vi "Temperature serial v6.vi"(0 "Command String":string, 5 "Time Out (S)":dbl, 7 "CALIB":dbl) -> (4 "T1":dbl, 6 "T2":dbl, 8 "T3":dbl, 10 "T4":dbl, 13 "error":bool, 14 "output cluster":cluster{dbl, dbl, dbl, dbl, i32, "error #":dbl}, 15 "Unit ID":dbl)   [LabVIEW 2013]
uses:
  program files/Global 1.vi
  <vilib>/Instr/_visa.llb/VISA Configure Serial Port (Instr).vi
panel:
  out "COM port":refnum<visa-resource-name>="COM6"
  out "error #":dbl
  out "End T":dbl
  out "Start T":dbl
  out "read time":dbl
  in  "Array - String":string[](array[string])
  out "end of data (#)":bool
  out "data bytes read":dbl
  out "data string":string
  out "read buffer":string
  out "error out":errorcluster
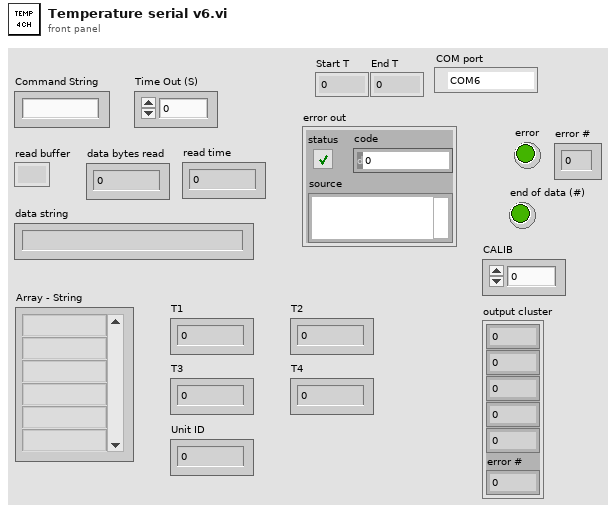
[diagram p1: front panel]
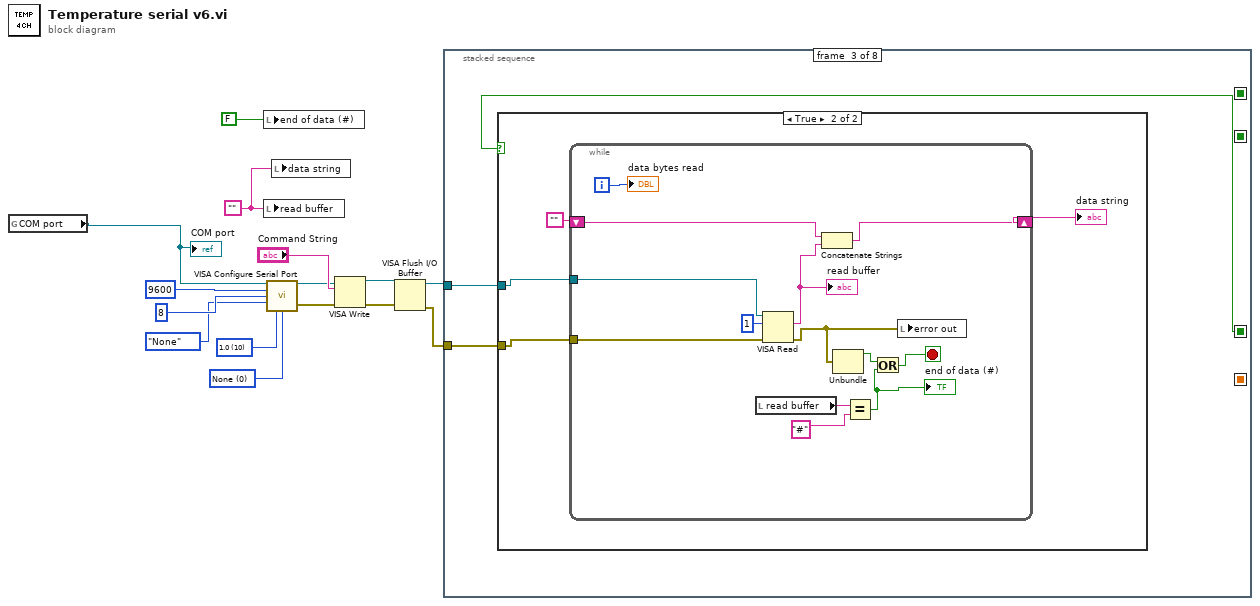
[diagram p0: block diagram]
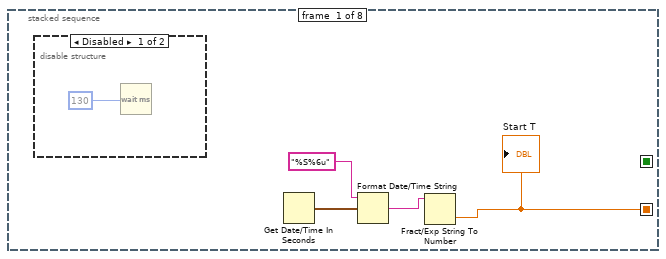
[diagram p2: hidden frame]
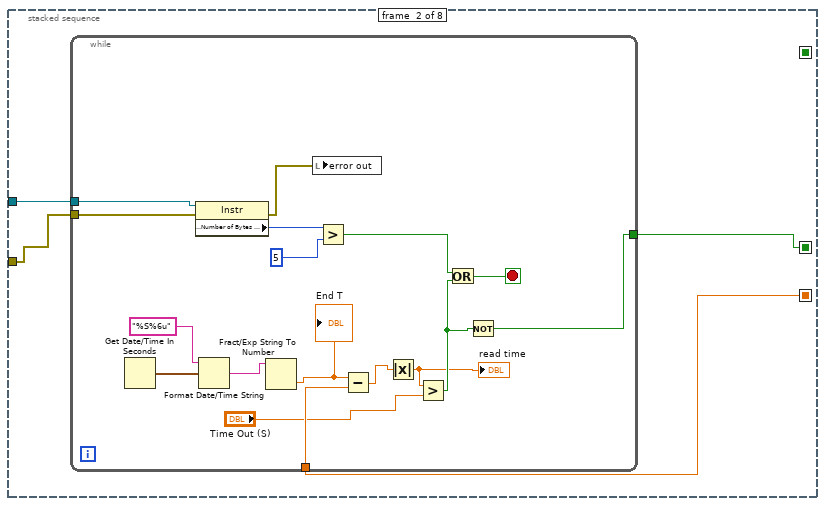
[diagram p4: hidden frame]
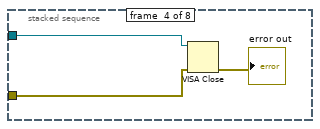
[diagram p6: hidden frame]
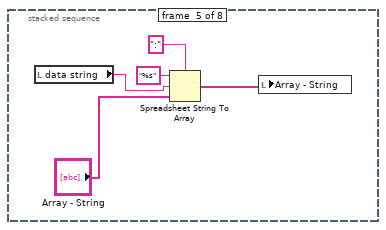
[diagram p7: hidden frame]
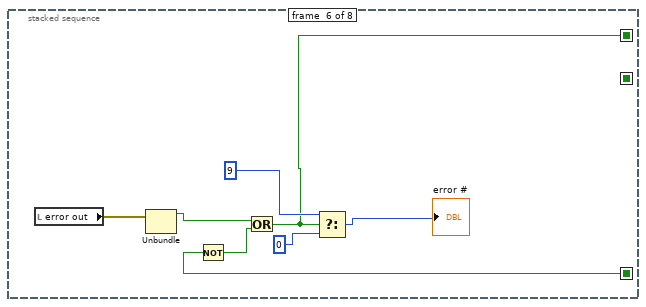
[diagram p8: hidden frame]
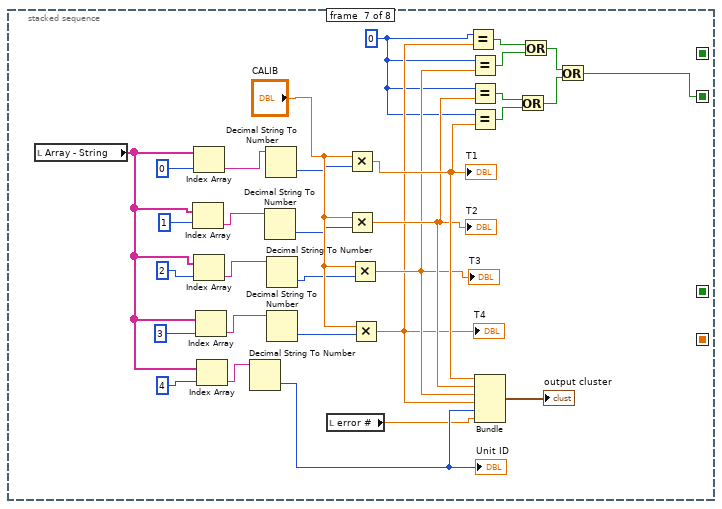
[diagram p9: hidden frame]
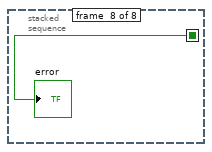
[diagram p10: hidden frame]
diagram:
  w2 = ""
  w11 = u16 0 items=["None", "XON/XOFF", "RTS/CTS", "XON/XOFF & RTS/CTS", "DTR/DSR", "XON/XOFF & DTR/DSR"] ("flow control (0:none)")
  w12 = u16 10 items=["1.0"=10, "1.5"=15, "2.0"=20] ("stop bits (10: 1 bit)")
  n1 = global read "Global 1.vi" "COM port"() -> (w1:refnum<visa-resource-name>)
  "COM port" <- w1
  n2 = local write "end of data (#)"(FALSE) -> ()
  n3 = local write "read buffer"(w2) -> ()
  n4 = call-poly "VISA Configure Serial Port"("VISA resource name"=w1, "baud rate (9600)"=u32 9600, "data bits (8)"=u16 8, "parity (0:none)"=enum16{"None", "Odd", "Even", "Mark", "Space"}."None", "stop bits (10: 1 bit)"=w12, "flow control (0:none)"=w11) -> ("VISA resource name out"=w4:refnum<visa-resource-name>, "error out"=w3:errorcluster)  [unwired: 8 in]
  n5 = local write "data string"(w2) -> ()
  n6 = VISA Write(VISA resource name=w4, write buffer="Command String", error in (no error)=w3) -> (VISA resource name out=w9:refnum<visa-resource-name>, error out=w8:errorcluster)  [unwired: 1 out]
  n7 = VISA Flush I/O Buffer(VISA resource name=w9, error in (no error)=w8) -> (VISA resource name out=w7:refnum<visa-resource-name>, error out=w6:errorcluster)  [unwired: 1 in]
  n8 = stacked-sequence {
    seq-local: [_ w22 _ _ _ _ _ _] -> [_ _ w42 _ _ w75 _ _]
    seq-local: [w16 _ _ _ _ _ _ _] -> [_ w21 _ _ _ _ _ _]
    seq-local: [_ _ _ _ _ w70 _ _] -> [_ _ _ _ _ _ _ _]
    seq-local: [_ _ _ _ _ _ w78 _] -> [_ _ _ _ _ _ _ w109]
    tunnel: w7 -> [_ w24 w44 w64 _ _ _ _]
    tunnel: w6 -> [_ w23 w43 w63 _ _ _ _]
    frame #0 {
      n9 = disable-structure shown="Disabled" {
        frame Disabled {
          n10 = Wait (ms)(milliseconds to wait=130) -> ()  [unwired: 1 out]
        }
        frame Enabled {
        }
      }
      n11 = Get Date/Time In Seconds() -> (seconds since 1Jan1904=w19:timestamp)
      n12 = Format Date/Time String(time format string (%c)="%S%6u", seconds (now)=w19) -> (date/time string=w17:string)  [unwired: 1 in]
      n13 = Fract/Exp String To Number(string=w17) -> (number=w16:dbl)  [unwired: 3 in, 1 out]
      "Start T" <- w16
    }
    frame #1 {
      n14 = while {
        tunnel: w24 -> [w41]
        tunnel: w23 -> [w40]
        tunnel: [w28] -> w22
        tunnel: w21 -> [w32]
        stop <- w30 stop-if-true
        n15 = Get Date/Time In Seconds() -> (seconds since 1Jan1904=w36:timestamp)
        n16 = property class="Instr"(reference=w41, error in=w40) -> (error out=w37:errorcluster, "Serial Settings:Number of Bytes at Serial Port"=w39:u32)  [unwired: 1 out]
        n17 = Format Date/Time String(time format string (%c)="%S%6u", seconds (now)=w36) -> (date/time string=w34:string)  [unwired: 1 in]
        n18 = Fract/Exp String To Number(string=w34) -> (number=w33:dbl)  [unwired: 3 in, 1 out]
        "End T" <- w33
        n19 = local write "error out"(w37) -> ()
        n20 = Greater?(x=w39, y=5) -> (0:w31:bool)
        n21 = Subtract(x=w33, y=w32) -> (x-y=w26:dbl)
        n22 = Absolute Value(x=w26) -> (abs(x)=w25:dbl)
        "read time" <- w25
        n23 = Greater?(x=w25, y="Time Out (S)") -> (0:w29:bool)
        n24 = Or(x=w31, y=w29) -> (x .or. y?=w30:bool)
        n25 = Not(x=w29) -> (.not. x?=w28:bool)
      }
    }
    frame #2 {
      n26 = case shown="True" w42 {
        tunnel: w44 -> [_ w48]
        tunnel: w43 -> [_ w47]
        frame False {
        }
        frame True {
          n27 = while {
            tunnel: w48 -> [w56]
            tunnel: w47 -> [w55]
            shift-right: [w54] -> w46
            shift-left: "" -> [w53]
            i -> [w57]
            stop <- w49 stop-if-true
            n28 = local read "read buffer"() -> (w60:string)
            n29 = VISA Read(VISA resource name=w56, byte count=u32 1, error in (no error)=w55) -> (read buffer=w58:string, error out=w52:errorcluster)  [unwired: 2 out]
            "read buffer" <- w58
            n30 = Concatenate Strings(w53, w58) -> (w54:string)
            n31 = Unbundle(w52) -> ("status"=w51:bool)  [unwired: 2 out]
            n32 = Equal?(x=w60, y="#") -> (x = y?=w50:bool)
            "end of data (#)" <- w50
            n33 = Or(x=w51, y=w50) -> (x .or. y?=w49:bool)
            n34 = local write "error out"(w52) -> ()
            "data bytes read" <- w57
          }
          "data string" <- w46
        }
      }
    }
    frame #3 {
      n35 = VISA Close(VISA resource name=w64, error in (no error)=w63) -> (error out=→"error out":errorcluster)
    }
    frame #4 {
      n36 = local read "data string"() -> (w67:string)
      n37 = Spreadsheet String To Array(delimiter (Tab)=":", format string="%s", spreadsheet string=w67, array type (2D Dbl)="Array - String") -> (array=w65:string[])
      n38 = local write "Array - String"(w65) -> ()
    }
    frame #5 {
      n39 = local read "error out"() -> (w77:errorcluster)
      n40 = Unbundle(w77) -> ("status"=w76:bool)  [unwired: 2 out]
      n41 = Not(x=w75) -> (.not. x?=w74:bool)
      n42 = Or(x=w76, y=w74) -> (x .or. y?=w70:bool)
      n43 = Select(t=9, s=w70, f=0) -> (s? t:f=→"error #":i32)
    }
    frame #6 {
      w85 = 0
      n44 = local read "Array - String"() -> (w100:string[])
      n45 = Index Array(array=w100, index=1) -> (element=w103:string)
      n46 = Index Array(array=w100, index=0) -> (element=w107:string)
      n47 = Index Array(array=w100, index=2) -> (element=w102:string)
      n48 = Index Array(array=w100, index=3) -> (element=w101:string)
      n49 = Index Array(array=w100, index=4) -> (element=w98:string)
      n50 = Decimal String To Number(string=w98) -> (number=w92:i32)  [unwired: 2 in, 1 out]
      "Unit ID" <- w92
      n51 = Decimal String To Number(string=w103) -> (number=w95:i32)  [unwired: 2 in, 1 out]
      n52 = Decimal String To Number(string=w107) -> (number=w96:i32)  [unwired: 2 in, 1 out]
      n53 = Decimal String To Number(string=w102) -> (number=w94:i32)  [unwired: 2 in, 1 out]
      n54 = Decimal String To Number(string=w101) -> (number=w93:i32)  [unwired: 2 in, 1 out]
      n55 = local read "error #"() -> (w91:dbl)
      n56 = Multiply(x="CALIB", y=w96) -> (x*y=w89:dbl)
      "T1" <- w89
      n57 = Multiply(x="CALIB", y=w95) -> (x*y=w88:dbl)
      "T2" <- w88
      n58 = Multiply(x="CALIB", y=w94) -> (x*y=w87:dbl)
      "T3" <- w87
      n59 = Multiply(x="CALIB", y=w93) -> (x*y=w86:dbl)
      "T4" <- w86
      n60 = Equal?(x=w85, y=w86) -> (x = y?=w81:bool)
      n61 = Equal?(x=w85, y=w87) -> (x = y?=w82:bool)
      n62 = Equal?(x=w85, y=w88) -> (x = y?=w84:bool)
      n63 = Equal?(x=w85, y=w89) -> (x = y?=w83:bool)
      n64 = Bundle(w89, w88, w87, w86, w92, "error #"=w91) -> (→"output cluster":cluster{dbl, dbl, dbl, dbl, i32, "error #":dbl})  [unwired: 1 in]
      n65 = Or(x=w84, y=w83) -> (x .or. y?=w79:bool)
      n66 = Or(x=w81, y=w82) -> (x .or. y?=w80:bool)
      n67 = Or(x=w80, y=w79) -> (x .or. y?=w78:bool)
    }
    frame #7 {
      "error" <- w109
    }
  }
